vi "WriteData.vi"(8 "error in (no error)":errorcluster, 9 "Data":variant, 10 "LogicName":string, 11 "PLC_Module in":refnum<class "PLC_Module.lvclass">) -> (0 "error out":errorcluster, 3 "PLC_Module out":refnum<class "PLC_Module.lvclass">)   [LabVIEW 2025, in "PLC_Module.lvlib" / "PLC_Module.lvclass"]
uses:
  PLC_Module.lvclass
  PLC_Module.lvclass/PLC_Module.ctl
  PLC_Abstr/PLC_Abstr Messages/Write Data Msg/Write Data Msg.lvclass/Write Data Msg.ctl
  <vilib>/ActorFramework/Message Enqueuer/Message Enqueuer.lvclass/Message Enqueuer.ctl
  Read Configuration.vi
  Read Connect.vi
  <vilib>/ActorFramework/Message Enqueuer/Enqueue.vi
  PLC_Abstr/PLC_Abstr Messages/Write Data Msg/Write Data Msg.lvclass
  C:/Program Files (x86)/National Instruments/LabVIEW 2025/vi.lib/ActorFramework/Message/Message.lvclass
  <vilib>/ActorFramework/Message Priority Queue/Priority Enqueue.vi
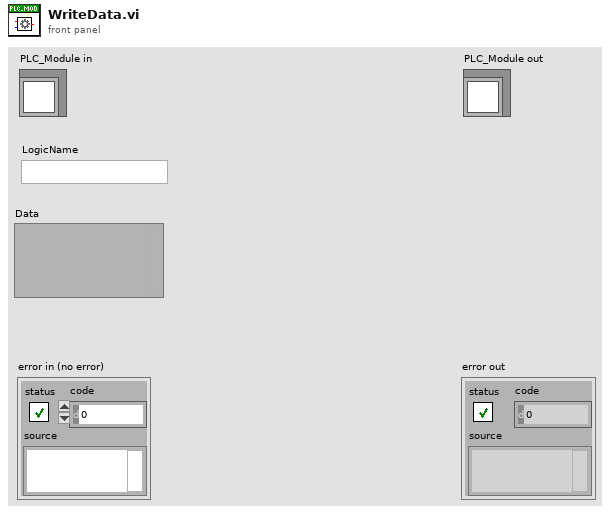
[diagram p1: front panel]
types:
  T1 = typedef "PLC_Module.lvlib/PLC_Module.lvclass/PLC_Data_Config.ctl" = map{string, cluster{"Config":T2, "Get Value":string, "Set Value":string}}
  T2 = typedef "PLC_Module.lvlib/PLC_Module.lvclass/PLC_Data.ctl" = cluster{"Address":string, "Direction":enum16{"PC->PLC", "PLC->PC"}, "DataType":T3, "Description":string}
  T3 = typedef "PLC_Module.lvlib/PLC_Module.lvclass/PLC_Data_Type.ctl" = enum16{"Boolean", "Single Float", "U8", "U32", "U32_Array", "String"}
  T4 = cluster{"Config":T2, "Get Value":string, "Set Value":string}
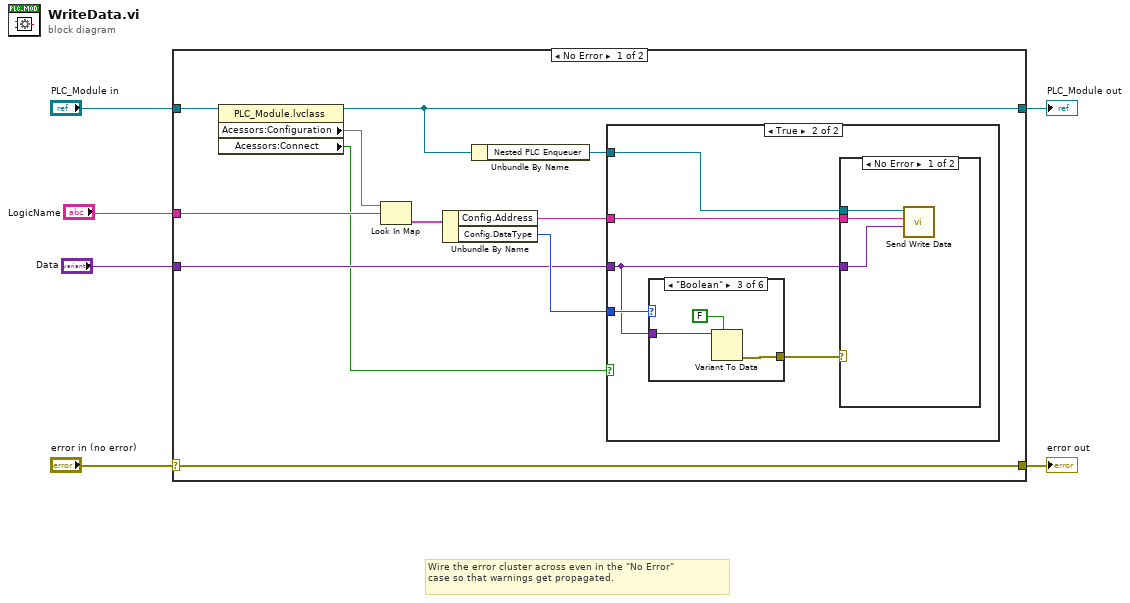
[diagram p0: block diagram]
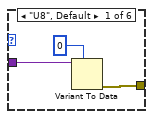
[diagram p4: hidden frame]
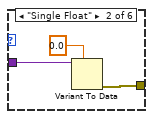
[diagram p5: hidden frame]
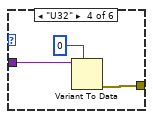
[diagram p6: hidden frame]
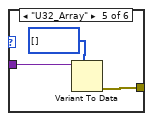
[diagram p7: hidden frame]
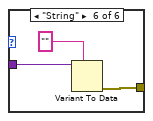
[diagram p8: hidden frame]
diagram:
  # "Wire the error cluster across even in the \"No Error\"\ncase so that warnings get propagated."
  n1 = case shown="No Error" "error in (no error)" {
    selector: "error in (no error)" -> [w16 w45]
    tunnel: [w16 w45] -> w5
    tunnel: [w13 w44] -> w3
    tunnel: "PLC_Module in" -> [w17 w44]
    tunnel: "LogicName" -> [w14 _]
    tunnel: "Data" -> [w8 _]
    frame No Error {
      n2 = property class="PLC_Module.lvclass"(reference=w17) -> (reference out=w13:refnum<class "PLC_Module.lvclass">, "Acessors:Configuration"=w15:T1, "Acessors:Connect"=w7:bool)  [unwired: 1 in, 1 out]
      n3 = Look In Map(map=w15, key=w14) -> (value=w11:T4)  [unwired: 1 in, 1 out]
      n4 = Unbundle By Name(w11) -> ("Config.Address"=w10:string, "Config.DataType"=w9:T3)
      n5 = Unbundle By Name(w13) -> ("Nested PLC Enqueuer"=w12:refnum<class "Message Enqueuer.lvclass">)
      n6 = case shown="True" w7 {
        tunnel: w12 -> [_ w22]
        tunnel: w10 -> [_ w21]
        tunnel: w9 -> [_ w20]
        tunnel: w8 -> [_ w18]
        frame False {
        }
        frame True {
          n7 = case shown="\"Boolean\"" w20 {
            tunnel: [w28 w31 w34 w37 w40 w43] -> w19
            tunnel: w18 -> [w27 w30 w33 w36 w39 w42]
            frame "U8", Default {
              n8 = Variant To Data(type=u8 0, Variant=w27) -> (error out=w28:errorcluster)  [unwired: 1 in, 1 out]
            }
            frame "Single Float" {
              n9 = Variant To Data(type=sgl 0.0, Variant=w30) -> (error out=w31:errorcluster)  [unwired: 1 in, 1 out]
            }
            frame "Boolean" {
              n10 = Variant To Data(type=FALSE, Variant=w33) -> (error out=w34:errorcluster)  [unwired: 1 in, 1 out]
            }
            frame "U32" {
              n11 = Variant To Data(type=u32 0, Variant=w36) -> (error out=w37:errorcluster)  [unwired: 1 in, 1 out]
            }
            frame "U32_Array" {
              n12 = Variant To Data(type=u32[] [], Variant=w39) -> (error out=w40:errorcluster)  [unwired: 1 in, 1 out]
            }
            frame "String" {
              n13 = Variant To Data(type="", Variant=w42) -> (error out=w43:errorcluster)  [unwired: 1 in, 1 out]
            }
          }
          n14 = case shown="No Error" w19 {
            tunnel: w22 -> [w25 _]
            tunnel: w21 -> [w24 _]
            tunnel: w18 -> [w23 _]
            frame No Error {
              n15 = call "Send Write Data.vi"("Data"=w23, "Address"=w24, "Message Enqueuer"=w25) -> ()  [unwired: 7 in, 2 out]
            }
            frame Error {
            }
          }
        }
      }
    }
    frame Error {
    }
  }
  "error out" <- w5
  "PLC_Module out" <- w3
